vi "Draw.vi"(7 "menu in":refnum<class "menu.lvclass">, 8 "error in (no error)":errorcluster, 11 "text in":refnum<class "text.lvclass">) -> (0 "error out":errorcluster, 3 "text out":refnum<class "text.lvclass">)   [LabVIEW 2009, in "text.lvclass"]
uses:
  text.lvclass
  Menu/menu.lvclass
  text.lvclass/text.ctl
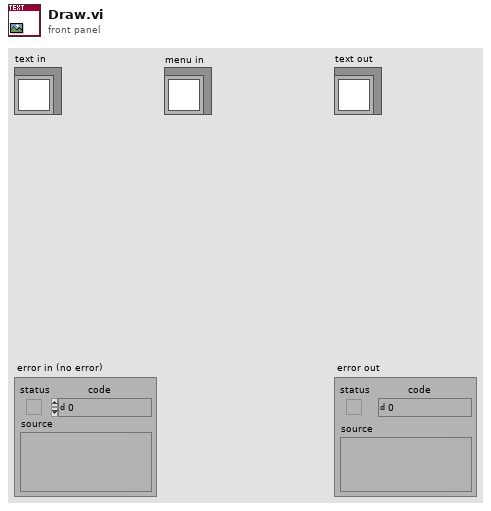
[diagram p1: front panel]
types:
  T1 = enum16{"Type?", "Plain", "Underline", "Parentheses", "End"}
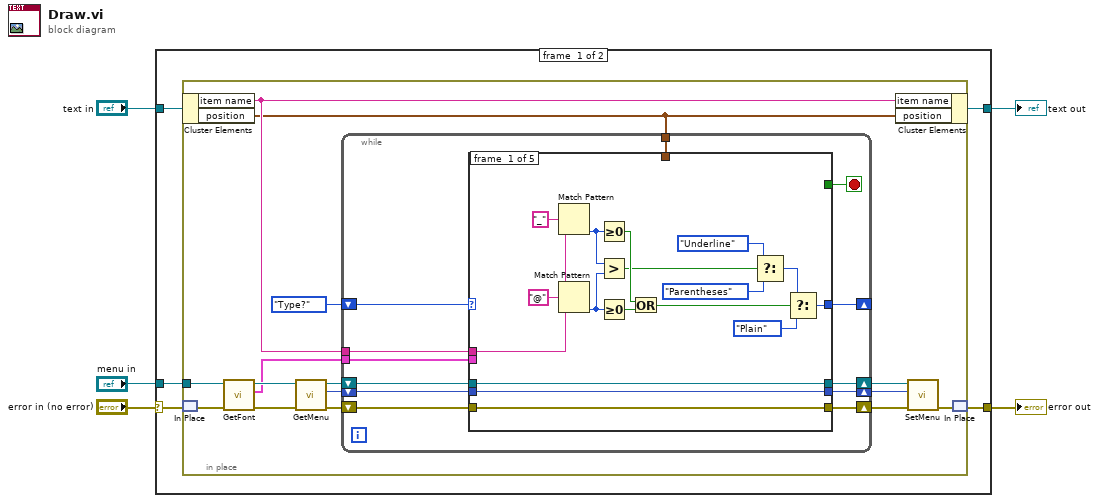
[diagram p0: block diagram]
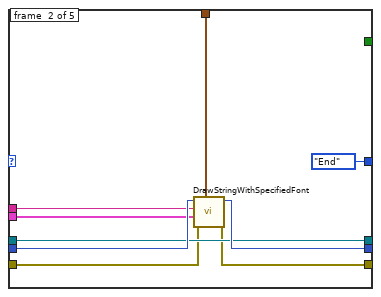
[diagram p2: hidden frame]
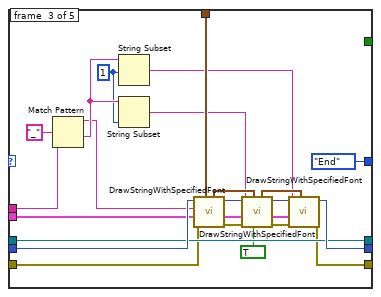
[diagram p3: hidden frame]
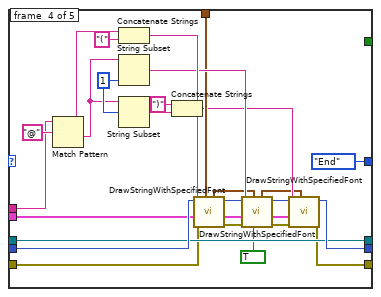
[diagram p4: hidden frame]
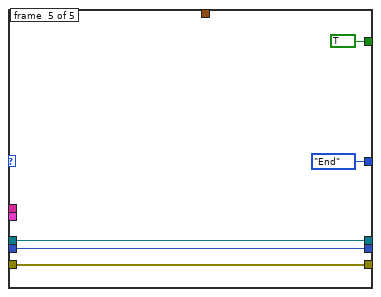
[diagram p5: hidden frame]
diagram:
  n1 = case shown="No Error" "error in (no error)" {
    selector: "error in (no error)" -> [w8 w118]
    tunnel: [w7 w118] -> w2
    tunnel: [w9 w117] -> w4
    tunnel: "text in" -> [w10 w117]
    tunnel: "menu in" -> [w6 _]
    frame #0 {
      n2 = in-place {
        in-place-border: w6 -> [w24]
        n3 = in-place-cluster #1(w10) -> ("item name"=w16:string, "position"=w11:cluster{"left":u32, "top":u32})
        n4 = in-place-match #2(w8) -> (w23:errorcluster)
        n5 = call "GetFont.vi"("error in (no error)"=w23, "menu in"=w24) -> ("error out"=w20:errorcluster, "font"=w12:cluster{"name":string, "size":i16, "color":u32}, "menu out"=w19:refnum<class "menu.lvclass">)  [unwired: 7 in]
        n6 = call "GetMenu.vi"("error in (no error)"=w20, "menu in"=w19) -> ("error out"=w17:errorcluster, "menu"=w21:picture, "menu out"=w14:refnum<class "menu.lvclass">)  [unwired: 7 in]
        n7 = while {
          shift-right: [w36] -> _
          shift-left: T1."Type?" ("state") -> [w37]
          tunnel: w16 -> [w35]
          shift-right: [w33] -> w22
          shift-left: w21 -> [w32]
          shift-right: [w28] -> w15
          shift-left: w17 -> [w31]
          shift-right: [w29] -> w13
          shift-left: w14 -> [w30]
          tunnel: w12 -> [w27]
          tunnel: w11 -> [w26]
          stop <- w34 stop-if-true
          n8 = case shown="\"Parentheses\"" w37 {
            tunnel: [w53 T1."End" ("state") T1."End" ("state") T1."End" ("state") T1."End" ("state")] -> w36
            tunnel: w35 -> [w38 w60 w83 w104 _]
            tunnel: [_ _ _ _ TRUE] -> w34
            tunnel: [w41 w63 w79 w101 w115] -> w33
            tunnel: w32 -> [w41 w62 w80 w100 w115]
            tunnel: w31 -> [w39 w59 w70 w90 w113]
            tunnel: w30 -> [w40 w61 w78 w99 w114]
            tunnel: [w40 w61 w78 w99 w114] -> w29
            tunnel: [w39 w58 w69 w91 w113] -> w28
            tunnel: w27 -> [_ w56 w71 w87 _]
            tunnel: w26 -> [_ w55 w73 w94 _]
            frame #0 {
              n9 = Match Pattern(string=w38, regular expression="_") -> (offset past match=w43:i32)  [unwired: 1 in, 3 out]
              n10 = Match Pattern(string=w38, regular expression="@") -> (offset past match=w42:i32)  [unwired: 1 in, 3 out]
              n11 = Greater Or Equal To 0?(x=w43) -> (x >= 0?=w47:bool)
              n12 = Greater?(x=w43, y=w42) -> (0:w44:bool)
              n13 = Greater Or Equal To 0?(x=w42) -> (x >= 0?=w48:bool)
              n14 = Or(x=w47, y=w48) -> (x .or. y?=w49:bool)
              n15 = Select(t=T1."Underline" ("state"), s=w44, f=T1."Parentheses" ("state")) -> (s? t:f=w50:T1)
              n16 = Select(t=w50, s=w49, f=T1."Plain" ("state")) -> (s? t:f=w53:T1)
            }
            frame #1 {
              n17 = call "DrawStringWithSpecifiedFont.vi"("position in"=w55, "error in (no error)"=w59, "font"=w56, "string"=w60, "picture in"=w62) -> ("error out"=w58:errorcluster, "picture out"=w63:picture)  [unwired: 4 in, 1 out]
            }
            frame #2 {
              w67 = 1 ("length (rest)")
              n18 = Match Pattern(string=w83, regular expression="_") -> (before substring=w72:string, after substring=w84:string)  [unwired: 1 in, 2 out]
              n19 = String Subset(string=w84, offset (0)=w67) -> (substring=w65:string)  [unwired: 1 in]
              n20 = String Subset(string=w84, length (rest)=w67) -> (substring=w66:string)  [unwired: 1 in]
              n21 = call "DrawStringWithSpecifiedFont.vi"("position in"=w73, "error in (no error)"=w70, "font"=w71, "string"=w72, "picture in"=w80) -> ("error out"=w77:errorcluster, "picture out"=w82:picture, "position out"=w75:cluster{"left":u32, "top":u32})  [unwired: 4 in]
              n22 = call "DrawStringWithSpecifiedFont.vi"("underline? (F)"=TRUE, "position in"=w75, "error in (no error)"=w77, "font"=w71, "string"=w66, "picture in"=w82) -> ("error out"=w76:errorcluster, "picture out"=w81:picture, "position out"=w74:cluster{"left":u32, "top":u32})  [unwired: 3 in]
              n23 = call "DrawStringWithSpecifiedFont.vi"("position in"=w74, "error in (no error)"=w76, "font"=w71, "string"=w65, "picture in"=w81) -> ("error out"=w69:errorcluster, "picture out"=w79:picture)  [unwired: 4 in, 1 out]
            }
            frame #3 {
              w110 = 1 ("length (rest)")
              n24 = Match Pattern(string=w104, regular expression="@") -> (before substring=w107:string, after substring=w108:string)  [unwired: 1 in, 2 out]
              n25 = Concatenate Strings(w107, "(" ("string")) -> (w96:string)
              n26 = String Subset(string=w108, length (rest)=w110) -> (substring=w95:string)  [unwired: 1 in]
              n27 = String Subset(string=w108, offset (0)=w110) -> (substring=w109:string)  [unwired: 1 in]
              n28 = Concatenate Strings(")" ("string"), w109) -> (w93:string)
              n29 = call "DrawStringWithSpecifiedFont.vi"("position in"=w94, "error in (no error)"=w90, "font"=w87, "string"=w96, "picture in"=w100) -> ("error out"=w98:errorcluster, "picture out"=w103:picture, "position out"=w89:cluster{"left":u32, "top":u32})  [unwired: 4 in]
              n30 = call "DrawStringWithSpecifiedFont.vi"("underline? (F)"=TRUE, "position in"=w89, "error in (no error)"=w98, "font"=w87, "string"=w95, "picture in"=w103) -> ("error out"=w97:errorcluster, "picture out"=w102:picture, "position out"=w88:cluster{"left":u32, "top":u32})  [unwired: 3 in]
              n31 = call "DrawStringWithSpecifiedFont.vi"("position in"=w88, "error in (no error)"=w97, "font"=w87, "string"=w93, "picture in"=w102) -> ("error out"=w91:errorcluster, "picture out"=w101:picture)  [unwired: 4 in, 1 out]
            }
            frame #4 {
            }
          }
        }
        n32 = in-place-cluster #1("item name"=w16, "position"=w11) -> (w9:refnum<class "text.lvclass">)
        n33 = call "SetMenu.vi"("error in (no error)"=w15, "menu"=w22, "menu in"=w13) -> ("error out"=w18:errorcluster)  [unwired: 7 in, 1 out]
        n34 = in-place-match #2(w18) -> (w7:errorcluster)
      }
    }
    frame #1 {
    }
  }
  "text out" <- w4
  "error out" <- w2
